vi "Convert Flow Rate.vi"(1 "Conversion":enum16{"Mass to Volume", "Volume to Mass"}(ring), 2 "P (mb)":dbl, 3 "T (K)":dbl, 4 "Qin":dbl) -> (0 "Qout":dbl)   [LabVIEW 2014]
doc: "Convert a mass flow to a volumetric flow or vice versa."
uses:
  Atmospheric/Atmospheric Constants.vi
  Atmospheric/Atmospheric Library.lvlib
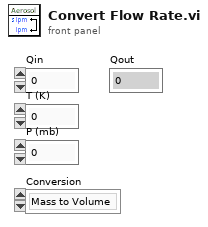
[diagram p1: front panel]
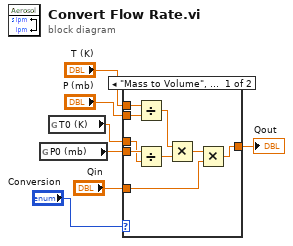
[diagram p0: block diagram]
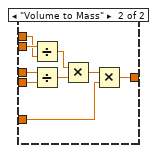
[diagram p2: hidden frame]
diagram:
  n1 = global read "Atmospheric Constants.vi" "P0 (mb)"() -> (w3:sgl)
  n2 = global read "Atmospheric Constants.vi" "T0 (K)"() -> (w2:sgl)
  n3 = case shown="\"Mass to Volume\", Default" "Conversion" {
    tunnel: "Qin" -> [w9 w18]
    tunnel: "T (K)" -> [w15 w22]
    tunnel: "P (mb)" -> [w16 w23]
    tunnel: w3 -> [w14 w25]
    tunnel: w2 -> [w13 w24]
    tunnel: [w8 w17] -> w1
    frame "Mass to Volume", Default {
      n4 = Divide(x=w15, y=w16) -> (x/y=w12:dbl)
      n5 = Divide(x=w14, y=w13) -> (x/y=w11:sgl)
      n6 = Multiply(x=w12, y=w11) -> (x*y=w10:dbl)
      n7 = Multiply(x=w10, y=w9) -> (x*y=w8:dbl)
    }
    frame "Volume to Mass" {
      n8 = Divide(x=w23, y=w22) -> (x/y=w20:dbl)
      n9 = Divide(x=w24, y=w25) -> (x/y=w21:sgl)
      n10 = Multiply(x=w20, y=w21) -> (x*y=w19:dbl)
      n11 = Multiply(x=w19, y=w18) -> (x*y=w17:dbl)
    }
  }
  "Qout" <- w1
